vi "AB_Source_Get_Property.vi"(8 "error in (no error)":errorcluster, 10 "type":T2, 11 "sourceProperties in":T1[](array[typedef])) -> (0 "error out":errorcluster, 1 "sourceProperty":T1={"sourcePropertyType"=enum."Password", "value"=variant}, 2 "found":bool, 3 "sourceProperties out":T1[](array[typedef]))   [LabVIEW 2020]
uses:
  <vilib>/AppBuilder/AB_Source_Properties.ctl
  <vilib>/AppBuilder/AB_Source_Property_Type.ctl
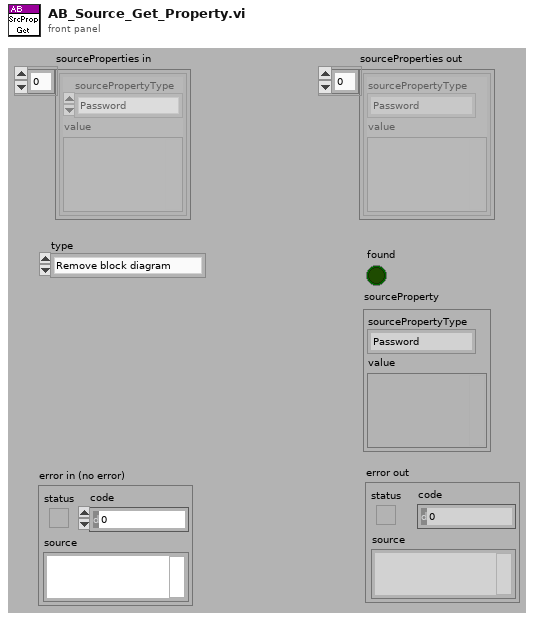
[diagram p1: front panel]
types:
  T1 = typedef "AB_Source_Properties.ctl" = cluster{"sourcePropertyType":T2, "value":variant}
  T2 = typedef "AB_Source_Property_Type.ctl" = enum16{"Remove block diagram", "Remove front panel", "Password", "Window has title bar", "Show menu bar", "Show vertical scroll bar", "Show horizontal scroll bar", "Show toolbar", "Show Abort button", "Show fp when called", "Window behavior", "Allow user to close window", "Window run-time position", "Run when opened", "Allow debugging", "Auto error handling", "Generate guard code", "Use stack variables", "Expression folding", "Integer only", "Inline subVI"}
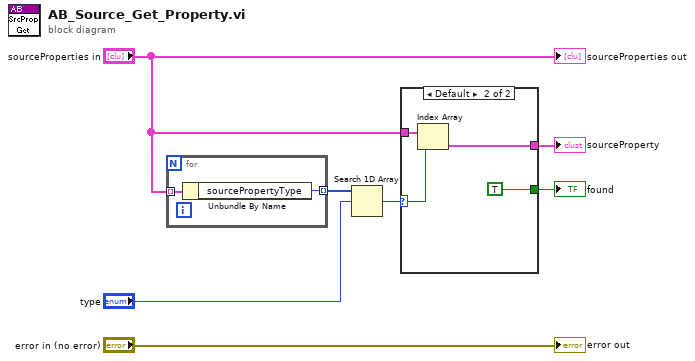
[diagram p0: block diagram]
diagram:
  n1 = for {
    tunnel: "sourceProperties in" -> [w9] mode=indexing
    tunnel: [w8] -> w7 mode=indexing
    n2 = Unbundle By Name(w9) -> ("sourcePropertyType"=w8:T2)
  }
  n3 = Search 1D Array(1D array=w7, element="type") -> (index of element=w5:i32)  [unwired: 1 in]
  n4 = case shown="Default" w5 {
    selector: w5 -> [_ w12]
    tunnel: "sourceProperties in" -> [_ w13]
    tunnel: [_ TRUE] -> w3
    tunnel: [_ w10] -> w1
    frame -1 {
    }
    frame Default {
      n5 = Index Array(array=w13, index=w12) -> (element=w10:T1)
    }
  }
  "found" <- w3
  "sourceProperty" <- w1
  "sourceProperties out" <- "sourceProperties in"
  "error out" <- "error in (no error)"
